vi "queueHandlerGlobals.vi"() -> ()   [LabVIEW 2014]
panel:
  out "DACQuWriteTimeout":bool
  out "MCSQuWriteTimeout":bool
  out "SPCtrQuWriteTimeout":bool
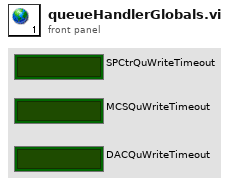
[diagram p1: front panel]
diagram:
